vi "delayedUI.vi"(7 "ms delay":u32=500, 8 "data":variant, 9 "message":string="quit", 11 "Queues in":T1) -> ()   [LabVIEW 2018]
uses:
  type defs/Queues.ctl
  Github/ICL-LabVIEW_General/Message Scheduler/generic message queue/standard message queue/standard message.lvclass
  supporting VIs/polymorphic VIs/enqueue for comms.vi
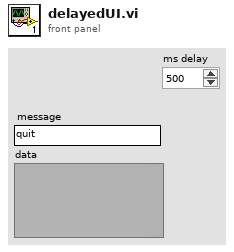
[diagram p1: front panel]
types:
  T1 = typedef "Queues.ctl" = cluster{"messageHandler":refnum<queue>, "comms":refnum<queue>, "dataStream":refnum<queue>, "dataProcessor":refnum<queue>, "fileIO":refnum<queue>, "userInterface":refnum<queue>, "errors":refnum<queue>, "customCompressor":refnum<queue>}
  T2 = cluster{"standard message out":refnum<class "standard message.lvclass">, "ms delay":u32}
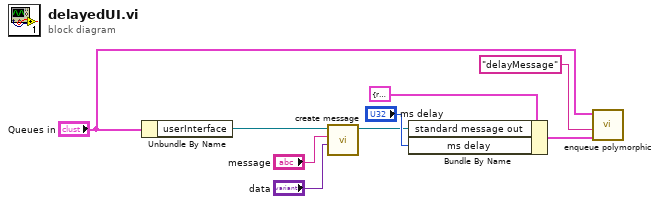
[diagram p0: block diagram]
diagram:
  n1 = Unbundle By Name("Queues in") -> ("userInterface"=w2:refnum<queue>)
  n2 = call "create message.vi"("data"="data", "message"="message", "queue ref"=w2) -> ("standard message out"=w6:refnum<class "standard message.lvclass">)  [unwired: 7 in, 1 out]
  n3 = Bundle By Name(cluster=T2 {"standard message out"=refnum, "ms delay"=1000}, "standard message out"=w6, "ms delay"="ms delay") -> (w8:T2)
  n4 = call-poly "enqueue polymorphic.vi"("data"=w8, "message"="delayMessage", "Queues"="Queues in") -> ()  [unwired: 8 in, 1 out]
